vi "Init PWM.vi"(5 "Phase-Correct (F)":bool, 7 "Enable (T)":bool=TRUE, 8 "error in (no error)":errorcluster, 10 "GPIO #":T1=-1, 11 "Session in":refnum<class "Session.lvclass">) -> (0 "error out":errorcluster, 3 "Session out":refnum<class "Session.lvclass">)   [LabVIEW 2024, in "CTI.lvlib" / "Session.lvclass"]
uses:
  Session.lvclass
  GPIO Number.ctl
  DeviceComms/DeviceComms.lvclass
  CTI.lvlib
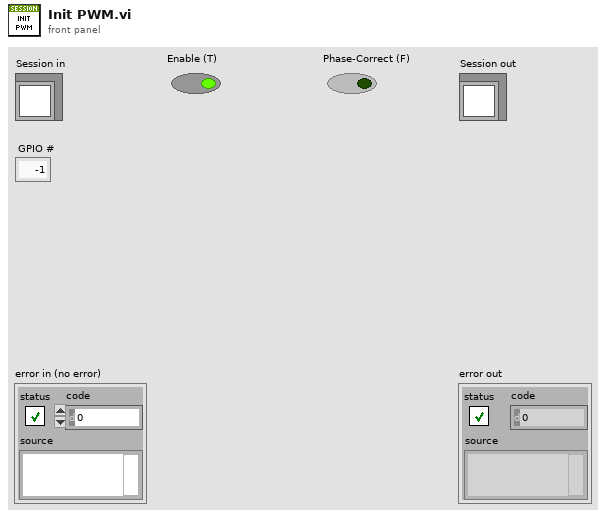
[diagram p1: front panel]
types:
  T1 = typedef "CTI.lvlib/GPIO Number.ctl" = i8
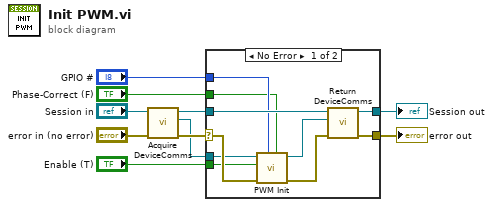
[diagram p0: block diagram]
diagram:
  n1 = call "Acquire DeviceComms.vi"("error in (no error)"="error in (no error)", "Session in"="Session in") -> ("error out"=w10:errorcluster, "DeviceComms"=w4:refnum<class "DeviceComms.lvclass">, "Session out"=w6:refnum<class "Session.lvclass">)  [unwired: 7 in]
  n2 = case shown="No Error" w10 {
    selector: w10 -> [w20 w22]
    tunnel: [w19 w22] -> w7
    tunnel: w6 -> [w18 w21]
    tunnel: [w17 w21] -> w5
    tunnel: w4 -> [w16 _]
    tunnel: "GPIO #" -> [w13 _]
    tunnel: "Phase-Correct (F)" -> [w12 _]
    tunnel: "Enable (T)" -> [w11 _]
    frame No Error {
      n3 = call-dynamic "PWM Init.vi"("Phase-Correct (F)"=w12, "GPIO #"=w13, "error in (no error)"=w20, "Enable (F)"=w11, "DeviceComms in"=w16) -> ("error out"=w14:errorcluster, "DeviceComms out"=w15:refnum<class "DeviceComms.lvclass">)  [unwired: 5 in]
      n4 = call "Return DeviceComms.vi"("error in (no error)"=w14, "DeviceComms"=w15, "Session in"=w18) -> ("error out"=w19:errorcluster, "Session out"=w17:refnum<class "Session.lvclass">)  [unwired: 7 in]
    }
    frame Error {
    }
  }
  "error out" <- w7
  "Session out" <- w5
